vi "OAT Gaussian Window.vi"(10 "standard\ndeviation":dbl format="%.2f", 11 "X":dbl[](array[numeric]) format="%.2f") -> (0 "error":i32, 2 "window constants":cluster{"eq noise BW":dbl, "coherent gain":dbl} {"coherent gain" format="%.2f"; "eq noise BW" format="%.2f"}, 3 "Y":dbl[](array[numeric]) format="%.2f")   [LabVIEW 2017]
panel:
  # "Gaussian Chirp Generator"
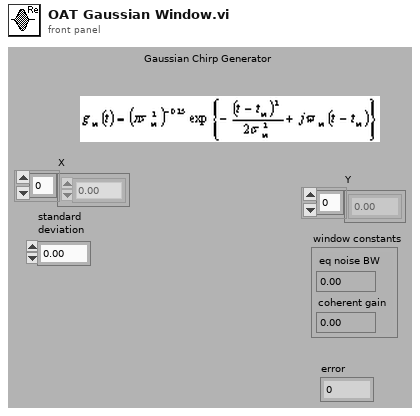
[diagram p1: front panel]
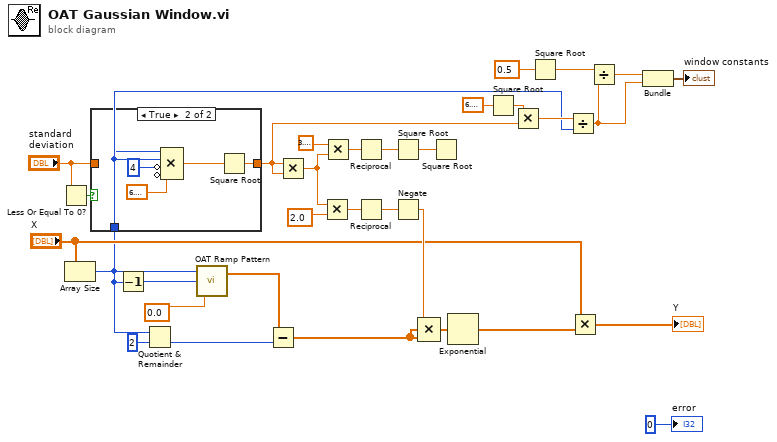
[diagram p0: block diagram]
diagram:
  n1 = Less Or Equal To 0?(x="standard\ndeviation") -> (x <= 0?=w16:bool)
  n2 = Array Size(array="X") -> (size(s)=w6:i32)
  n3 = case shown="True" w16 {
    tunnel: w6 -> [_ w37]
    tunnel: [w33 w38] -> w9
    tunnel: "standard\ndeviation" -> [w33 _]
    frame False {
    }
    frame True {
      n4 = Compound Arithmetic op=MULTIPLY(w37, w37, invert 4 ("value"), invert 6.283185307179586) -> (w34:dbl)
      n5 = Square Root(x=w34) -> (sqrt(x)=w38:dbl)
    }
  }
  n6 = Decrement(x=w6) -> (x-1=w30:i32)
  n7 = Quotient & Remainder(x=w6, y=2) -> (floor(x/y)=w18:i32)  [unwired: 1 out]
  n8 = call <vilib>:"OAT Ramp Pattern.vi"("start"=0.0, "end"=w30, "samples"=w6) -> ("Ramp Pattern"=w22:dbl[])  [unwired: 1 out]
  n9 = Subtract(x=w22, y=w18) -> (x-y=w12:dbl[])
  n10 = Multiply(x=w9, y=w9) -> (x*y=w20:dbl)
  n11 = Multiply(x=w20, y=2.0 ("Input")) -> (x*y=w26:dbl)
  n12 = Multiply(x=3.141592653589793, y=w20) -> (x*y=w25:dbl)
  n13 = Reciprocal(x=w25) -> (1/x=w24:dbl)
  n14 = Reciprocal(x=w26) -> (1/x=w31:dbl)
  n15 = Square Root(x=w24) -> (sqrt(x)=w23:dbl)
  n16 = Negate(x=w31) -> (-x=w28:dbl)
  n17 = Compound Arithmetic op=MULTIPLY(w28, w12, w12) -> (w15:dbl[])
  n18 = Square Root(x=w23) -> ()  [unwired: 1 out]
  n19 = Exponential(1:w15) -> (0:w7:dbl[])
  n20 = Square Root(x=6.283185307179586) -> (sqrt(x)=w10:dbl)
  n21 = Multiply(x=w10, y=w9) -> (x*y=w8:dbl)
  n22 = Square Root(x=0.5 ("Input")) -> (sqrt(x)=w4:dbl)
  n23 = Divide(x=w8, y=w6) -> (x/y=w2:dbl)
  n24 = Multiply(x="X", y=w7) -> (x*y=→"Y":dbl[])
  n25 = Divide(x=w4, y=w2) -> (x/y=w3:dbl)
  n26 = Bundle(w3, w2) -> (→"window constants":cluster{dbl, dbl})  [unwired: 1 in]
  "error" <- 0
